vi "Main On Compile Action VI_Parse BC.vi"(7 "Autocreate Rx timestamp chans?":bool, 8 "error in":errorcluster, 10 "Channel Ref":u64, 11 "Device Item Ref in":T2 format="%.0x") -> (0 "error out":errorcluster, 2 "Channel Ref":u64, 3 "BC":T1 {"Acyclic Frames Trigger Channels Refs" format="%.0x"; "Command Channels Refs" format="%.0x"; "messages"."Timestamp Channel Data Reference" format="%.0x"; "messages"."Status Channel Data Refs" format="%.0x"; "messages"."Words Item Refs" format="%.0x"; "messages"."Words Block Data Refs"."Data Reference" format="%.0x"})   [LabVIEW 2020, in "Ballard 1553 System Explorer.lvlib"]
uses:
  Ballard 1553 System Explorer.lvlib
  <vilib>/NI VeriStand/Custom Device API/Custom Device Item Ref.ctl
  Shared/Controls and Global/RT BC.ctl
  Shared/Controls and Global/RT Message.ctl
  Shared/Controls and Global/RT messageType.ctl
  Shared/Controls and Global/RT CWD1.ctl
  Shared/Controls and Global/RT CWD2.ctl
  <vilib>/NI VeriStand/Custom Device API/Data Reference.ctl
  <vilib>/NI VeriStand/Custom Device API/Block Data Reference.ctl
  Shared/EncodeDecode/_typedefs/parameter_config_type.ctl
  Shared/EncodeDecode/_typedefs/parameter_config_type_type.ctl
  Shared/EncodeDecode/_typedefs/parameter_config_encoding_type.ctl
  Parse XML Ballard/Ballard_messageType.ctl
  Parse XML Ballard/Ballard_CWD1.ctl
  Parse XML Ballard/Ballard_CWD2.ctl
  <vilib>/NI VeriStand/Custom Device API/Data Access Type.ctl
  Shared/Controls and Global/Global.vi
  <vilib>/NI VeriStand/Custom Device Tools/Custom Device Utility Library/NI VeriStand - Search for Item by GUID.vi
  <vilib>/NI VeriStand/Custom Device API/Get Item Property (I32).vi
  <vilib>/NI VeriStand/Custom Device API/Get Item Property (String).vi
  <vilib>/NI VeriStand/Custom Device Tools/Custom Device Utility Library/NI VeriStand - Search for Item by Name.vi
  <vilib>/NI VeriStand/Custom Device Tools/Custom Device Utility Library/NI VeriStand - Search for All Items by GUID.vi
  <vilib>/NI VeriStand/Custom Device API/Get Item Property (Variant).vi
  <vilib>/NI VeriStand/Custom Device API/Get Item Property (U16).vi
  Shared/Ballard 1553 Shared.lvlib
  <vilib>/NI VeriStand/Custom Device Tools/Custom Device Utility Library/Custom Device Utility Library.lvlib
  <vilib>/NI VeriStand/Custom Device API/Custom Device API.lvlib
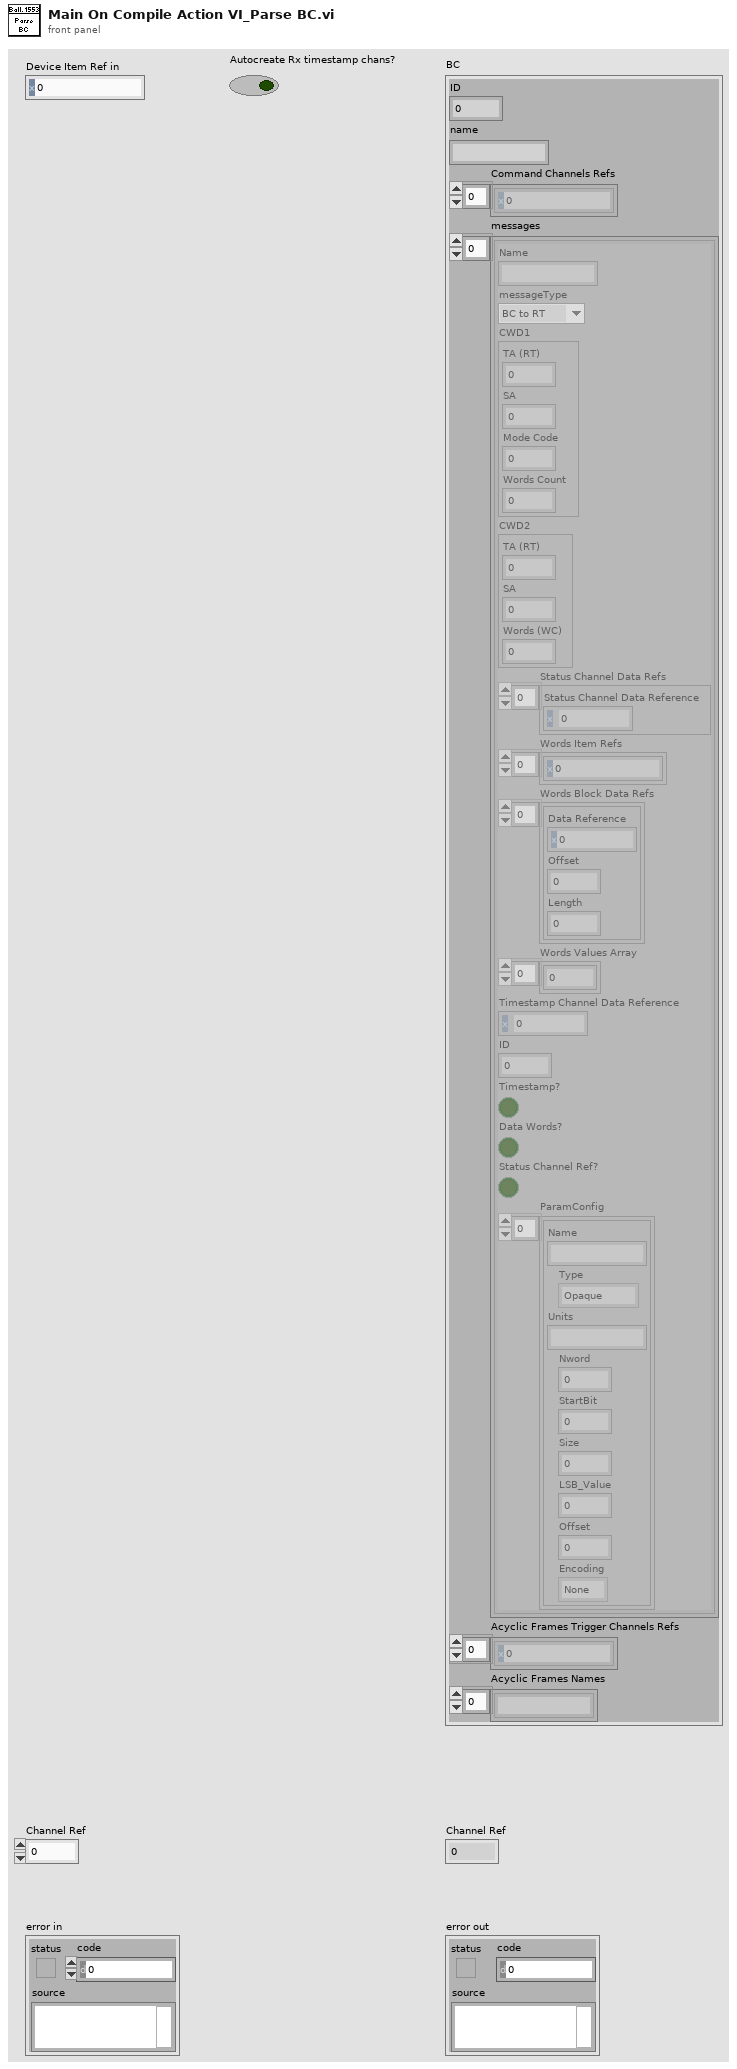
[diagram p1: front panel]
types:
  T1 = typedef "Ballard 1553 Shared.lvlib/RT BC.ctl" = cluster{"ID":i32, "name":string, "Command Channels Refs":T2[], "messages":T3[], "Acyclic Frames Trigger Channels Refs":T2[], "Acyclic Frames Names":string[]}
  T2 = typedef "Custom Device API.lvlib/Custom Device Item Ref.ctl" = u64
  T3 = typedef "Ballard 1553 Shared.lvlib/RT Message.ctl" = cluster{"Name":string, "messageType":T4, "CWD1":T5, "CWD2":T6, "Status Channel Data Refs":T7[], "Words Item Refs":T2[], "Words Block Data Refs":T8[], "Words Values Array":u16[], "Timestamp Channel Data Reference":T7, "ID":i32, "Timestamp?":bool, "Data Words?":bool, "Status Channel Ref?":bool, "ParamConfig":T9[]}
  T4 = typedef "Ballard 1553 Shared.lvlib/RT messageType.ctl" = enum16{"BC to RT", "RT to BC", "RT to RT", "MC (Rx)", "MC (Tx)"}
  T5 = typedef "Ballard 1553 Shared.lvlib/RT CWD1.ctl" = cluster{"TA (RT)":i8, "SA":i8, "Mode Code":i8, "Words Count":i8}
  T6 = typedef "Ballard 1553 Shared.lvlib/RT CWD2.ctl" = cluster{"TA (RT)":i8, "SA":i8, "Words (WC)":i8}
  T7 = typedef "Custom Device API.lvlib/Data Reference.ctl" = i32
  T8 = typedef "Custom Device API.lvlib/Block Data Reference.ctl" = cluster{"Data Reference":T7, "Offset":u64, "Length":u64}
  T9 = typedef "parameter_config_type.ctl" = cluster{"Name":string, "Type":T10, "Units":string, "Nword":i32, "StartBit":i32, "Size":i32, "LSB_Value":i32, "Offset":i32, "Encoding":T11}
  T10 = typedef "parameter_config_type_type.ctl" = enum16{"Opaque", "Enum", "Float", "Integer", "Bcd", "Bool"}
  T11 = typedef "parameter_config_encoding_type.ctl" = enum16{"None", "2-complement", "Unsigned"}
  T12 = typedef "Ballard 1553 System Explorer.lvlib/Ballard_CWD2.ctl" = cluster{"TA (RT)":i8, "SA":i8, "Words (WC)":i8}
  T13 = typedef "Ballard 1553 System Explorer.lvlib/Ballard_CWD1.ctl" = cluster{"TA (RT)":i8, "SA":i8, "Mode Code":i8, "Words Count":i8}
  T14 = typedef "Ballard 1553 System Explorer.lvlib/Ballard_messageType.ctl" = enum16{"BC to RT", "RT to BC", "RT to RT", "MC (Rx)", "MC (Tx)"}
  T15 = typedef "Custom Device API.lvlib/Data Access Type.ctl" = enum16{"Read", "Write"}
  T16 = typedef "Custom Device API.lvlib/Custom Device Item Info.ctl" = cluster{"Name":string, "Is Channel":bool, "GUID":string, "Is Waveform":bool}
  T17 = typedef "Custom Device API.lvlib/Custom Device Channel.ctl" = cluster{"Type":T18, "Units":string, "Default Value":dbl, "Faultable":bool, "Scalable":bool}
  T18 = typedef "Custom Device API.lvlib/Custom Device Channel Type.ctl" = enum16{"Input", "Output"}
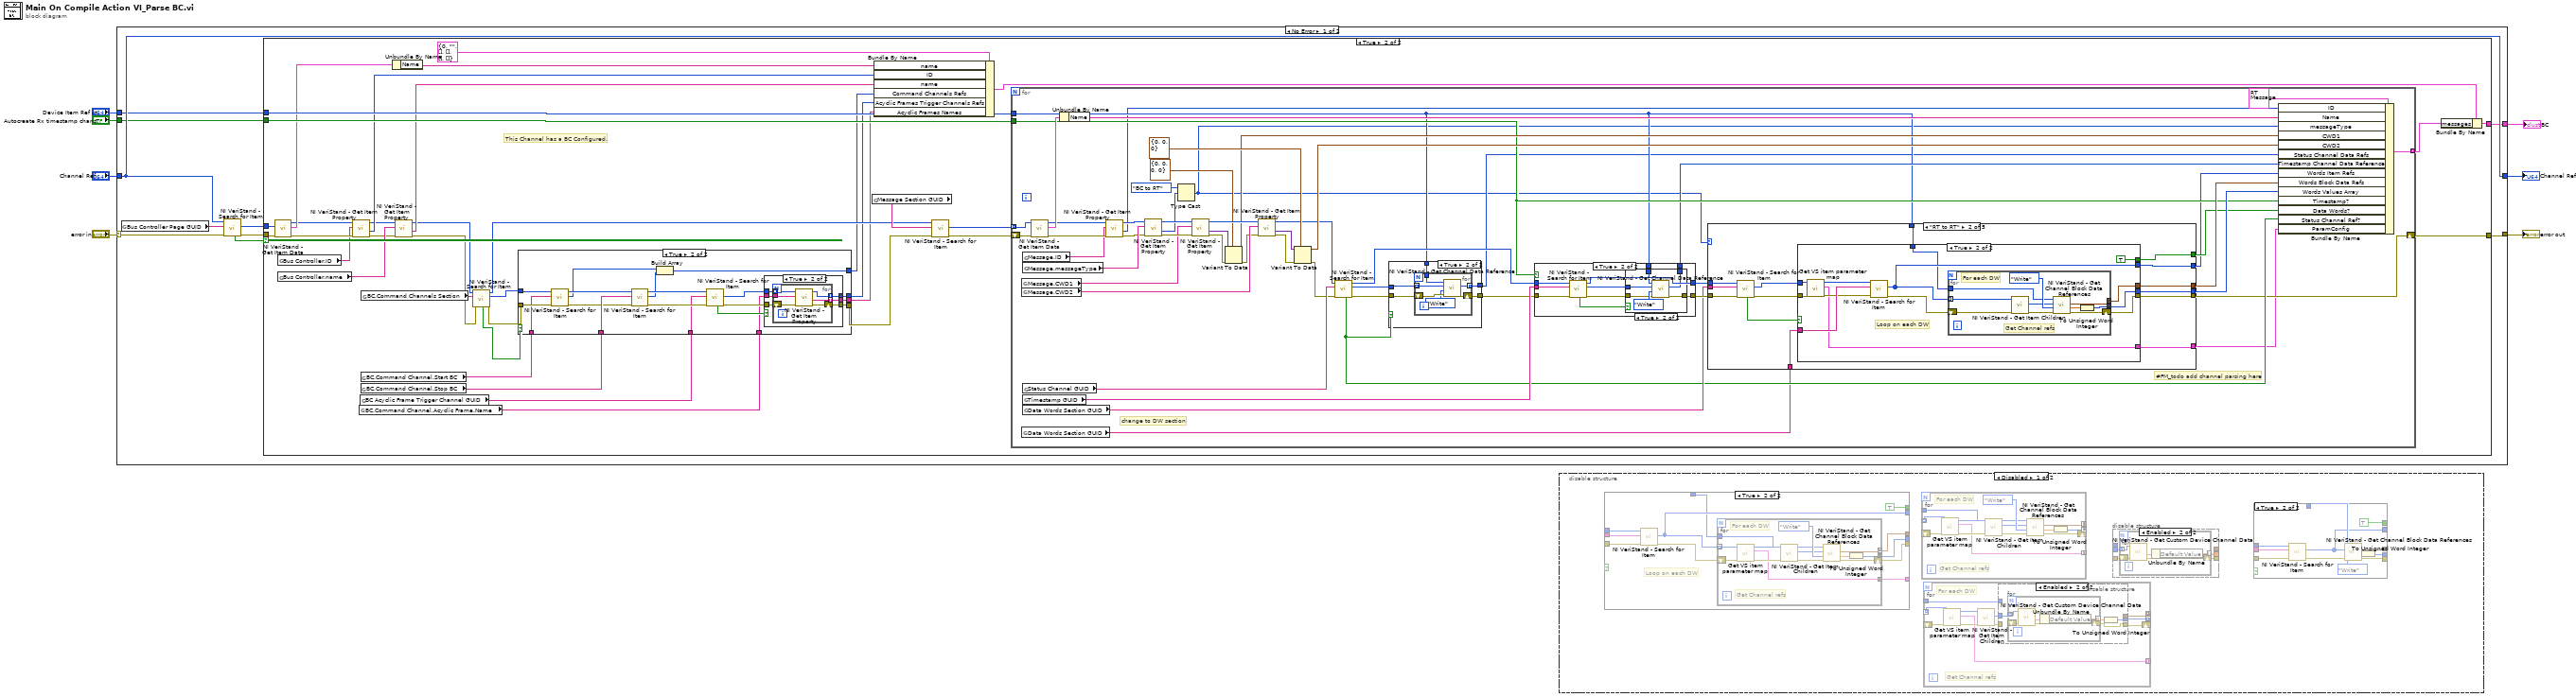
[diagram p0: block diagram]
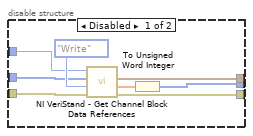
[diagram p2: hidden frame]
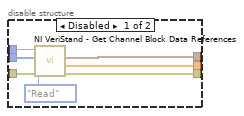
[diagram p3: hidden frame]
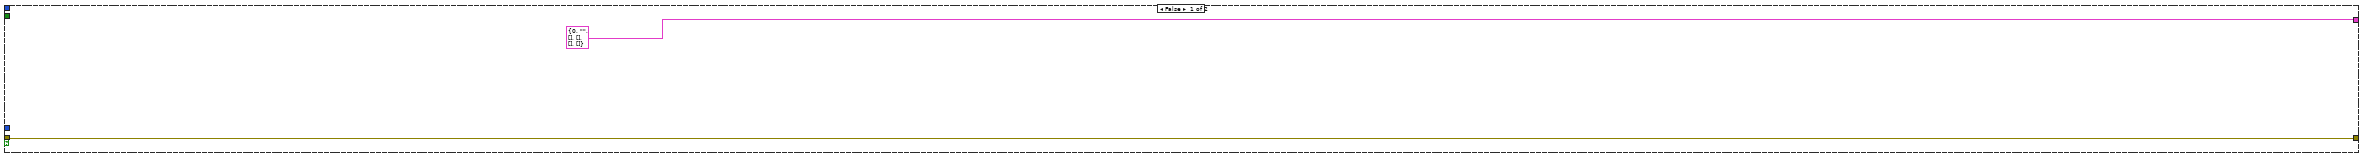
[diagram p7: hidden frame]
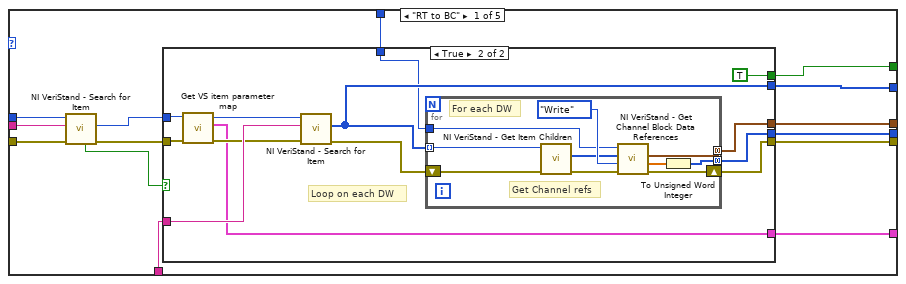
[diagram p11: hidden frame]
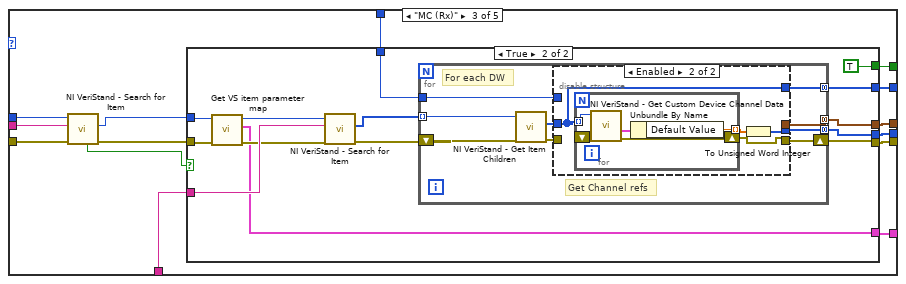
[diagram p14: hidden frame]
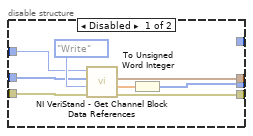
[diagram p16: hidden frame]
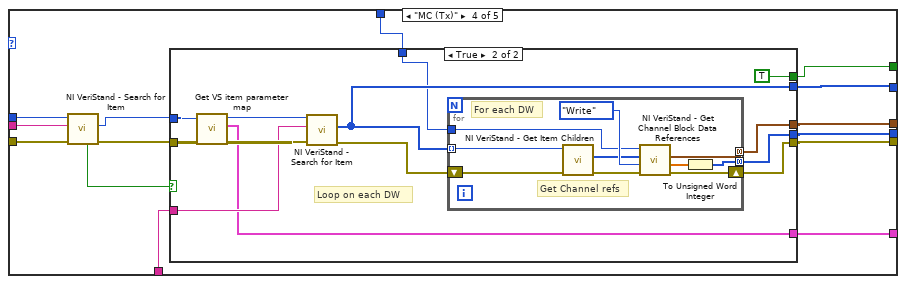
[diagram p17: hidden frame]
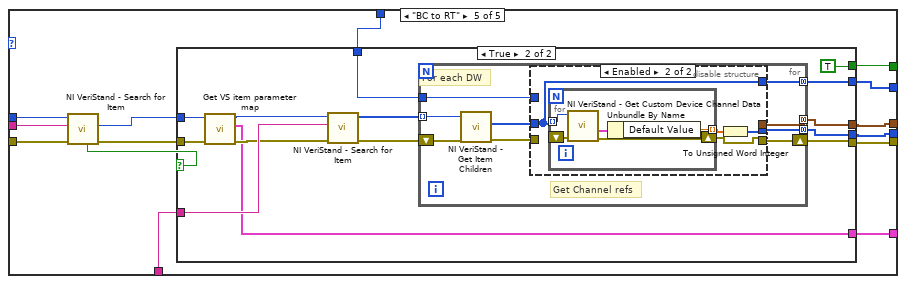
[diagram p19: hidden frame]
diagram:
  n1 = case shown="No Error" "error in" {
    selector: "error in" -> [w16 w401]
    tunnel: [w17 w401] -> w6
    tunnel: "Channel Ref" -> [w14 w400]
    tunnel: [w14 w400] -> w4
    tunnel: "Autocreate Rx timestamp chans?" -> [w10 _]
    tunnel: "Device Item Ref in" -> [w9 _]
    tunnel: [w8 T1 {"ID"=0, "name"="", "Command Channels Refs"=[], "messages"=[], "Acyclic Frames Trigger Channels Refs"=[], "Acyclic Frames Names"=[]} ("BC")] -> w1
    frame No Error {
      n2 = global read "Global.vi" "Bus Controller Page GUID"() -> (w15:string)
      n3 = call-poly <vilib>:"NI VeriStand - Search for Item.vi"("error in"=w16, "Item GUID"=w15, "Section Ref in"=w14) -> ("error out"=w13:errorcluster, "Item Ref"=w11:T2, "Found"=w12:bool)  [unwired: 5 in, 1 out]
      n4 = case shown="True" w12 {
        tunnel: w13 -> [w19 w39]
        tunnel: w11 -> [_ w40]
        tunnel: w10 -> [_ w53]
        tunnel: [w19 w52] -> w17
        tunnel: w9 -> [_ w51]
        tunnel: [T1 {"ID"=0, "name"="", "Command Channels Refs"=[], "messages"=[], "Acyclic Frames Trigger Channels Refs"=[], "Acyclic Frames Names"=[]} ("BC") w49] -> w8
        frame False {
        }
        frame True {
          # "This Channel has a BC Configured."
          n5 = call <vilib>:"NI VeriStand - Get Item Data.vi"("error in (no error)"=w39, "Item Ref in"=w40) -> ("error out"=w33:errorcluster, "Item Info"=w38:T16, "Item Ref out"=w34:T2)  [unwired: 6 in, 1 out]
          n6 = global read "Global.vi" "Bus Controller.ID"() -> (w32:string)
          n7 = global read "Global.vi" "Bus Controller.name"() -> (w29:string)
          n8 = call-poly <vilib>:"NI VeriStand - Get Item Property.vi"("error in (no error)"=w33, "Property Name"=w32, "Item Ref in"=w34) -> ("error out"=w28:errorcluster, "Value"=w31:i32, "Item Ref out"=w30:T2)  [unwired: 5 in, 1 out]
          n9 = global read "Global.vi" "BC.Command Channel.Acyclic Frame.Name"() -> (w22:string)
          n10 = global read "Global.vi" "BC Acyclic Frame Trigger Channel GUID"() -> (w23:string)
          n11 = global read "Global.vi" "BC.Command Channel.Start BC"() -> (w43:string)
          n12 = global read "Global.vi" "BC.Command Channel.Stop BC"() -> (w42:string)
          n13 = global read "Global.vi" "BC.Command Channels Section"() -> (w45:string)
          n14 = Unbundle By Name(w38) -> ("Name"=w36:string)
          n15 = call-poly <vilib>:"NI VeriStand - Get Item Property.vi"("error in (no error)"=w28, "Property Name"=w29, "Item Ref in"=w30) -> ("error out"=w27:errorcluster, "Value"=w26:string, "Item Ref out"=w24:T2)  [unwired: 5 in, 1 out]
          n16 = call-poly <vilib>:"NI VeriStand - Search for Item.vi"("error in"=w27, "Item Name"=w45, "Section Ref in"=w24) -> ("error out"=w46:errorcluster, "Item Ref"=w48:T2, "Section Ref out"=w41:T2, "Found"=w47:bool)  [unwired: 5 in]
          n17 = case shown="True" w47 {
            tunnel: w46 -> [w57 w76]
            tunnel: w48 -> [_ w75]
            tunnel: w43 -> [_ w74]
            tunnel: w42 -> [_ w73]
            tunnel: [w57 w61] -> w44
            tunnel: [_ w70] -> w25
            tunnel: [_ w60] -> w21
            tunnel: w23 -> [_ w68]
            tunnel: [_ w59] -> w20
            tunnel: w22 -> [_ w58]
            frame False {
            }
            frame True {
              n18 = call-poly <vilib>:"NI VeriStand - Search for Item.vi"("error in"=w76, "Item Name"=w74, "Section Ref in"=w75) -> ("error out"=w71:errorcluster, "Item Ref"=w66:T2, "Section Ref out"=w72:T2)  [unwired: 5 in, 1 out]
              n19 = call-poly <vilib>:"NI VeriStand - Search for Item.vi"("error in"=w71, "Item Name"=w73, "Section Ref in"=w72) -> ("error out"=w69:errorcluster, "Item Ref"=w65:T2, "Section Ref out"=w67:T2)  [unwired: 5 in, 1 out]
              n20 = Build Array(w66, w65) -> (w70:T2[])
              n21 = call-poly <vilib>:"NI VeriStand - Search for Item.vi"("error in"=w69, "Item GUID"=w68, "Section Ref in"=w67) -> ("error out"=w63:errorcluster, "Item Refs"=w62:T2[], "Found"=w64:bool)  [unwired: 5 in, 1 out]
              n22 = case shown="True" w64 {
                tunnel: w63 -> [w78 w83]
                tunnel: w62 -> [w77 w84]
                tunnel: [w78 w82] -> w61
                tunnel: [w77 w81] -> w60
                tunnel: [_ w80] -> w59
                tunnel: w58 -> [_ w79]
                frame False {
                }
                frame True {
                  n23 = for {
                    tunnel: w84 -> [w90] mode=indexing
                    shift-right: [w88] -> w82
                    shift-left: w83 -> [w89]
                    tunnel: [w87] -> w81 mode=indexing
                    tunnel: [w86] -> w80 mode=indexing
                    tunnel: w79 -> [w85]
                    n24 = call-poly <vilib>:"NI VeriStand - Get Item Property.vi"("error in (no error)"=w89, "Property Name"=w85, "Item Ref in"=w90) -> ("error out"=w88:errorcluster, "Value"=w86:string, "Item Ref out"=w87:T2)  [unwired: 5 in, 1 out]
                  }
                }
              }
            }
          }
          n25 = global read "Global.vi" "Message Section GUID"() -> (w56:string)
          n26 = Bundle By Name(cluster=T1 {"ID"=0, "name"="", "Command Channels Refs"=[], "messages"=[], "Acyclic Frames Trigger Channels Refs"=[], "Acyclic Frames Names"=[]} ("BC"), "name"=w36, "ID"=w31, "name"=w26, "Command Channels Refs"=w25, "Acyclic Frames Trigger Channels Refs"=w21, "Acyclic Frames Names"=w20) -> (w35:T1)
          n27 = call-poly <vilib>:"NI VeriStand - Search for Item.vi"("error in"=w44, "Item GUID"=w56, "Section Ref in"=w41) -> ("error out"=w55:errorcluster, "Item Refs"=w54:T2[])  [unwired: 5 in, 2 out]
          n28 = for {
            tunnel: w54 -> [w122] mode=indexing
            shift-right: [w94] -> w52
            shift-left: w55 -> [w123]
            tunnel: w53 -> [w106]
            tunnel: w51 -> [w98]
            tunnel: [w115] -> w50 mode=indexing
            # "change to DW section"
            # "#FM_todo add channel parsing here"
            n29 = global read "Global.vi" "Message.CWD1"() -> (w139:string)
            n30 = global read "Global.vi" "Message.CWD2"() -> (w138:string)
            n31 = global read "Global.vi" "Data Words Section GUID"() -> (w93:string)
            n32 = global read "Global.vi" "Message.ID"() -> (w109:string)
            n33 = global read "Global.vi" "Message.messageType"() -> (w140:string)
            n34 = global read "Global.vi" "Status Channel GUID"() -> (w128:string)
            n35 = global read "Global.vi" "Timestamp GUID"() -> (w127:string)
            n36 = global read "Global.vi" "Data Words Section GUID"() -> (w124:string)
            n37 = call <vilib>:"NI VeriStand - Get Item Data.vi"("error in (no error)"=w123, "Item Ref in"=w122) -> ("error out"=w110:errorcluster, "Item Info"=w121:T16, "Item Ref out"=w111:T2)  [unwired: 6 in, 1 out]
            n38 = Unbundle By Name(w121) -> ("Name"=w120:string)
            n39 = call-poly <vilib>:"NI VeriStand - Get Item Property.vi"("error in (no error)"=w110, "Property Name"=w109, "Item Ref in"=w111) -> ("error out"=w108:errorcluster, "Value"=w95:i32, "Item Ref out"=w107:T2)  [unwired: 5 in, 1 out]
            n40 = call-poly <vilib>:"NI VeriStand - Get Item Property.vi"("error in (no error)"=w108, "Property Name"=w140, "Item Ref in"=w107) -> ("error out"=w143:errorcluster, "Value"=w132:u16, "Item Ref out"=w141:T2)  [unwired: 5 in, 1 out]
            n41 = Type Cast(type=Ballard_messageType."BC to RT" ("messageType"), x=w132) -> (*(type *) &x=w96:T14)
            n42 = call-poly <vilib>:"NI VeriStand - Get Item Property.vi"("error in (no error)"=w143, "Property Name"=w139, "Item Ref in"=w141) -> ("error out"=w137:errorcluster, "Value"=w134:variant, "Item Ref out"=w142:T2)  [unwired: 5 in, 1 out]
            n43 = Variant To Data(error in=w137, type=T13 {"TA (RT)"=0, "SA"=0, "Mode Code"=0, "Words Count"=0} ("CWD1"), Variant=w134) -> (data=w119:T13, error out=w135:errorcluster)
            n44 = call-poly <vilib>:"NI VeriStand - Get Item Property.vi"("error in (no error)"=w135, "Property Name"=w138, "Item Ref in"=w142) -> ("error out"=w136:errorcluster, "Value"=w133:variant, "Item Ref out"=w114:T2)  [unwired: 5 in, 1 out]
            n45 = Variant To Data(error in=w136, type=T12 {"TA (RT)"=0, "SA"=0, "Words (WC)"=0} ("CWD1"), Variant=w133) -> (data=w118:T12, error out=w113:errorcluster)
            n46 = call-poly <vilib>:"NI VeriStand - Search for Item.vi"("error in"=w113, "Item GUID"=w128, "Section Ref in"=w114) -> ("error out"=w102:errorcluster, "Item Refs"=w100:T2[], "Section Ref out"=w99:T2, "Found"=w103:bool)  [unwired: 5 in]
            n47 = case shown="True" w103 {
              tunnel: w102 -> [w144 w149]
              tunnel: [w144 w148] -> w101
              tunnel: w100 -> [_ w146]
              tunnel: w98 -> [_ w147]
              tunnel: [_ w145] -> w97
              frame False {
              }
              frame True {
                n48 = for {
                  tunnel: w147 -> [w153]
                  shift-right: [w154] -> w148
                  shift-left: w149 -> [w155]
                  tunnel: w146 -> [w151] mode=indexing
                  tunnel: [w150] -> w145 mode=indexing
                  n49 = call <vilib>:"NI VeriStand - Get Channel Data Reference.vi"("error in (no error)"=w155, "Access"=Data_Access_Type."Write", "Channel Ref in"=w151, "Device Ref in"=w153) -> ("error out"=w154:errorcluster, "Channel Data Reference"=w150:T7)  [unwired: 5 in, 1 out]
                }
              }
            }
            n50 = case shown="True" w106 {
              tunnel: w99 -> [w380 w391]
              tunnel: w101 -> [w381 w390]
              tunnel: [w381 w388] -> w126
              tunnel: w127 -> [_ w389]
              tunnel: [w380 w386] -> w125
              tunnel: w98 -> [_ w385]
              tunnel: [_ w383] -> w104
              frame False {
              }
              frame True {
                n51 = call-poly <vilib>:"NI VeriStand - Search for Item.vi"("error in"=w390, "Item GUID"=w389, "Section Ref in"=w391) -> ("error out"=w387:errorcluster, "Item Ref"=w384:T2, "Section Ref out"=w386:T2, "Found"=w382:bool)  [unwired: 5 in]
                n52 = case shown="True" w382 {
                  tunnel: [w392 w397] -> w388
                  tunnel: w387 -> [w392 w396]
                  tunnel: w385 -> [_ w395]
                  tunnel: w384 -> [_ w394]
                  tunnel: [_ w393] -> w383
                  frame False {
                  }
                  frame True {
                    n53 = call <vilib>:"NI VeriStand - Get Channel Data Reference.vi"("error in (no error)"=w396, "Access"=Data_Access_Type."Write", "Channel Ref in"=w394, "Device Ref in"=w395) -> ("error out"=w397:errorcluster, "Channel Data Reference"=w393:T7)  [unwired: 5 in, 1 out]
                  }
                }
              }
            }
            n54 = case shown="\"RT to RT\"" w96 {
              tunnel: w126 -> [w169 w207 w245 w300 w338]
              tunnel: w125 -> [w168 w206 w244 w299 w337]
              tunnel: w124 -> [w167 w205 w243 w298 w336]
              tunnel: w93 -> [w164 w203 w239 w295 w333]
              tunnel: [w163 w197 w238 w290 w328] -> w94
              tunnel: w98 -> [w162 w200 w237 w293 w331]
              tunnel: [w161 w198 w236 w292 w329] -> w117
              tunnel: [w160 w199 w235 w291 w330] -> w116
              tunnel: [w159 w196 w233 w288 w326] -> w92
              tunnel: [w158 w195 w234 w289 w327] -> w105
              tunnel: [w156 w194 w232 w287 w335] -> w91
              frame "RT to BC" {
                n55 = call-poly <vilib>:"NI VeriStand - Search for Item.vi"("error in"=w169, "Item GUID"=w167, "Section Ref in"=w168) -> ("error out"=w166:errorcluster, "Item Ref"=w165:T2, "Found"=w157:bool)  [unwired: 5 in, 1 out]
                n56 = case shown="True" w157 {
                  tunnel: w166 -> [w170 w174]
                  tunnel: w165 -> [_ w175]
                  tunnel: w164 -> [_ w183]
                  tunnel: [w170 w176] -> w163
                  tunnel: w162 -> [_ w179]
                  tunnel: [_ w180] -> w159
                  tunnel: [_ w177] -> w161
                  tunnel: [_ w178] -> w160
                  tunnel: [_ TRUE] -> w158
                  tunnel: [_ w171] -> w156
                  frame False {
                  }
                  frame True {
                    # "Loop on each DW"
                    n57 = call "Get VS item parameter map.vi"("error in (no error)"=w174, "Iten refs in"=w175) -> ("error out"=w173:errorcluster, "param config out"=w171:T9[], "Iten refs out"=w172:T2)  [unwired: 6 in, 1 out]
                    n58 = call-poly <vilib>:"NI VeriStand - Search for Item.vi"("error in"=w173, "Item GUID"=w183, "Section Ref in"=w172) -> ("error out"=w181:errorcluster, "Item Refs"=w180:T2[])  [unwired: 5 in, 2 out]
                    n59 = for {
                      shift-right: [w188] -> w176
                      shift-left: w181 -> [w186]
                      tunnel: w180 -> [w187] mode=indexing
                      tunnel: w179 -> [w191]
                      tunnel: [w190] -> w178 mode=concatenating
                      tunnel: [w189] -> w177 mode=concatenating
                      # "Get Channel refs"
                      # "For each DW"
                      n60 = call <vilib>:"NI VeriStand - Get Item Children.vi"("error in (no error)"=w186, "Item Ref in"=w187) -> ("error out"=w184:errorcluster, "Child Refs"=w185:T2[])  [unwired: 6 in, 2 out]
                      n61 = call <vilib>:"NI VeriStand - Get Channel Block Data References.vi"("error in (no error)"=w184, "Access"=Data_Access_Type."Write", "Channel Refs"=w185, "Device Ref in"=w191) -> ("error out"=w188:errorcluster, "Values Array"=w193:dbl[], "Block Data Refs"=w189:T8[])  [unwired: 4 in, 1 out]
                      n62 = To Unsigned Word Integer(number=w193) -> (unsigned 16bit integer=w190:u16[])
                    }
                  }
                }
              }
              frame "RT to RT" {
                n63 = call-poly <vilib>:"NI VeriStand - Search for Item.vi"("error in"=w207, "Item GUID"=w205, "Section Ref in"=w206) -> ("error out"=w202:errorcluster, "Item Ref"=w204:T2, "Found"=w201:bool)  [unwired: 5 in, 1 out]
                n64 = case shown="True" w201 {
                  tunnel: w202 -> [w208 w212]
                  tunnel: w204 -> [_ w213]
                  tunnel: w203 -> [_ w221]
                  tunnel: [w208 w214] -> w197
                  tunnel: w200 -> [_ w217]
                  tunnel: [_ w218] -> w196
                  tunnel: [_ w215] -> w198
                  tunnel: [_ w216] -> w199
                  tunnel: [_ TRUE] -> w195
                  tunnel: [_ w209] -> w194
                  frame False {
                  }
                  frame True {
                    # "Loop on each DW"
                    n65 = call "Get VS item parameter map.vi"("error in (no error)"=w212, "Iten refs in"=w213) -> ("error out"=w211:errorcluster, "param config out"=w209:T9[], "Iten refs out"=w210:T2)  [unwired: 6 in, 1 out]
                    n66 = call-poly <vilib>:"NI VeriStand - Search for Item.vi"("error in"=w211, "Item GUID"=w221, "Section Ref in"=w210) -> ("error out"=w219:errorcluster, "Item Refs"=w218:T2[])  [unwired: 5 in, 2 out]
                    n67 = for {
                      shift-right: [w226] -> w214
                      shift-left: w219 -> [w224]
                      tunnel: w218 -> [w225] mode=indexing
                      tunnel: w217 -> [w229]
                      tunnel: [w228] -> w216 mode=concatenating
                      tunnel: [w227] -> w215 mode=concatenating
                      # "Get Channel refs"
                      # "For each DW"
                      n68 = call <vilib>:"NI VeriStand - Get Item Children.vi"("error in (no error)"=w224, "Item Ref in"=w225) -> ("error out"=w222:errorcluster, "Child Refs"=w223:T2[])  [unwired: 6 in, 2 out]
                      n69 = call <vilib>:"NI VeriStand - Get Channel Block Data References.vi"("error in (no error)"=w222, "Access"=Data_Access_Type."Write", "Channel Refs"=w223, "Device Ref in"=w229) -> ("error out"=w226:errorcluster, "Values Array"=w231:dbl[], "Block Data Refs"=w227:T8[])  [unwired: 4 in, 1 out]
                      n70 = To Unsigned Word Integer(number=w231) -> (unsigned 16bit integer=w228:u16[])
                    }
                  }
                }
              }
              frame "MC (Rx)" {
                n71 = call-poly <vilib>:"NI VeriStand - Search for Item.vi"("error in"=w245, "Item GUID"=w243, "Section Ref in"=w244) -> ("error out"=w242:errorcluster, "Item Ref"=w240:T2, "Found"=w241:bool)  [unwired: 5 in, 1 out]
                n72 = case shown="True" w241 {
                  tunnel: w242 -> [w246 w251]
                  tunnel: w240 -> [_ w250]
                  tunnel: w239 -> [_ w260]
                  tunnel: [w246 w256] -> w238
                  tunnel: w237 -> [_ w253]
                  tunnel: [_ w255] -> w236
                  tunnel: [_ w254] -> w235
                  tunnel: [_ TRUE] -> w234
                  tunnel: [_ w252] -> w233
                  tunnel: [_ w247] -> w232
                  frame False {
                  }
                  frame True {
                    n73 = call "Get VS item parameter map.vi"("error in (no error)"=w251, "Iten refs in"=w250) -> ("error out"=w248:errorcluster, "param config out"=w247:T9[], "Iten refs out"=w249:T2)  [unwired: 6 in, 1 out]
                    n74 = call-poly <vilib>:"NI VeriStand - Search for Item.vi"("error in"=w248, "Item GUID"=w260, "Section Ref in"=w249) -> ("error out"=w257:errorcluster, "Item Refs"=w258:T2[])  [unwired: 5 in, 2 out]
                    n75 = for {
                      shift-right: [w266] -> w256
                      shift-left: w257 -> [w264]
                      tunnel: w258 -> [w265] mode=indexing
                      tunnel: w253 -> [w269]
                      tunnel: [w268] -> w254 mode=concatenating
                      tunnel: [w267] -> w255 mode=concatenating
                      tunnel: [w261] -> w252 mode=concatenating
                      # "Get Channel refs"
                      # "For each DW"
                      n76 = call <vilib>:"NI VeriStand - Get Item Children.vi"("error in (no error)"=w264, "Item Ref in"=w265) -> ("error out"=w262:errorcluster, "Child Refs"=w263:T2[])  [unwired: 6 in, 2 out]
                      n77 = disable-structure shown="Enabled" {
                        disable-tunnel: w269 -> [w275 _]
                        disable-tunnel: [w274 w280] -> w268
                        disable-tunnel: [w273 _] -> w267
                        disable-tunnel: [w272 w279] -> w266
                        disable-tunnel: w263 -> [w271 w278]
                        disable-tunnel: w262 -> [w270 _]
                        disable-tunnel: [_ w278] -> w261
                        frame Disabled {
                          n78 = call <vilib>:"NI VeriStand - Get Channel Block Data References.vi"("error in (no error)"=w270, "Access"=Data_Access_Type."Write", "Channel Refs"=w271, "Device Ref in"=w275) -> ("error out"=w272:errorcluster, "Values Array"=w277:dbl[], "Block Data Refs"=w273:T8[])  [unwired: 4 in, 1 out]
                          n79 = To Unsigned Word Integer(number=w277) -> (unsigned 16bit integer=w274:u16[])
                        }
                        frame Enabled {
                          n80 = for {
                            tunnel: [w282] -> w281 mode=indexing
                            shift-right: [w283] -> w279
                            shift-left: _ -> [w286]
                            tunnel: w278 -> [w284] mode=indexing
                            n81 = call <vilib>:"NI VeriStand - Get Custom Device Channel Data.vi"("error in (no error)"=w286, "Channel Ref in"=w284) -> ("error out"=w283:errorcluster, "Channel"=w285:T17)  [unwired: 4 in, 4 out]
                            n82 = Unbundle By Name(w285) -> ("Default Value"=w282:dbl)
                          }
                          n83 = To Unsigned Word Integer(number=w281) -> (unsigned 16bit integer=w280:u16[])
                        }
                      }
                    }
                  }
                }
              }
              frame "MC (Tx)" {
                n84 = call-poly <vilib>:"NI VeriStand - Search for Item.vi"("error in"=w300, "Item GUID"=w298, "Section Ref in"=w299) -> ("error out"=w297:errorcluster, "Item Ref"=w294:T2, "Found"=w296:bool)  [unwired: 5 in, 1 out]
                n85 = case shown="True" w296 {
                  tunnel: w297 -> [w301 w305]
                  tunnel: w294 -> [_ w306]
                  tunnel: w295 -> [_ w314]
                  tunnel: [w301 w307] -> w290
                  tunnel: w293 -> [_ w310]
                  tunnel: [_ w311] -> w288
                  tunnel: [_ w308] -> w292
                  tunnel: [_ w309] -> w291
                  tunnel: [_ TRUE] -> w289
                  tunnel: [_ w302] -> w287
                  frame False {
                  }
                  frame True {
                    # "Loop on each DW"
                    n86 = call "Get VS item parameter map.vi"("error in (no error)"=w305, "Iten refs in"=w306) -> ("error out"=w303:errorcluster, "param config out"=w302:T9[], "Iten refs out"=w304:T2)  [unwired: 6 in, 1 out]
                    n87 = call-poly <vilib>:"NI VeriStand - Search for Item.vi"("error in"=w303, "Item GUID"=w314, "Section Ref in"=w304) -> ("error out"=w312:errorcluster, "Item Refs"=w311:T2[])  [unwired: 5 in, 2 out]
                    n88 = for {
                      shift-right: [w319] -> w307
                      shift-left: w312 -> [w317]
                      tunnel: w311 -> [w318] mode=indexing
                      tunnel: w310 -> [w322]
                      tunnel: [w321] -> w309 mode=concatenating
                      tunnel: [w320] -> w308 mode=concatenating
                      # "Get Channel refs"
                      # "For each DW"
                      n89 = call <vilib>:"NI VeriStand - Get Item Children.vi"("error in (no error)"=w317, "Item Ref in"=w318) -> ("error out"=w315:errorcluster, "Child Refs"=w316:T2[])  [unwired: 6 in, 2 out]
                      n90 = call <vilib>:"NI VeriStand - Get Channel Block Data References.vi"("error in (no error)"=w315, "Access"=Data_Access_Type."Write", "Channel Refs"=w316, "Device Ref in"=w322) -> ("error out"=w319:errorcluster, "Values Array"=w324:dbl[], "Block Data Refs"=w320:T8[])  [unwired: 4 in, 1 out]
                      n91 = To Unsigned Word Integer(number=w324) -> (unsigned 16bit integer=w321:u16[])
                    }
                  }
                }
              }
              frame "BC to RT" {
                n92 = call-poly <vilib>:"NI VeriStand - Search for Item.vi"("error in"=w338, "Item GUID"=w336, "Section Ref in"=w337) -> ("error out"=w334:errorcluster, "Item Ref"=w332:T2, "Found"=w325:bool)  [unwired: 5 in, 1 out]
                n93 = case shown="True" w325 {
                  tunnel: w334 -> [w339 w343]
                  tunnel: w332 -> [_ w344]
                  tunnel: w333 -> [_ w353]
                  tunnel: [w339 w349] -> w328
                  tunnel: w331 -> [_ w346]
                  tunnel: [_ w348] -> w329
                  tunnel: [_ w347] -> w330
                  tunnel: [_ TRUE] -> w327
                  tunnel: [_ w340] -> w335
                  tunnel: [_ w345] -> w326
                  frame False {
                  }
                  frame True {
                    n94 = call "Get VS item parameter map.vi"("error in (no error)"=w343, "Iten refs in"=w344) -> ("error out"=w342:errorcluster, "param config out"=w340:T9[], "Iten refs out"=w341:T2)  [unwired: 6 in, 1 out]
                    n95 = call-poly <vilib>:"NI VeriStand - Search for Item.vi"("error in"=w342, "Item GUID"=w353, "Section Ref in"=w341) -> ("error out"=w350:errorcluster, "Item Refs"=w351:T2[])  [unwired: 5 in, 2 out]
                    n96 = for {
                      shift-right: [w359] -> w349
                      shift-left: w350 -> [w357]
                      tunnel: w351 -> [w358] mode=indexing
                      tunnel: w346 -> [w362]
                      tunnel: [w361] -> w347 mode=concatenating
                      tunnel: [w360] -> w348 mode=concatenating
                      tunnel: [w354] -> w345 mode=concatenating
                      # "Get Channel refs"
                      # "For each DW"
                      n97 = call <vilib>:"NI VeriStand - Get Item Children.vi"("error in (no error)"=w357, "Item Ref in"=w358) -> ("error out"=w355:errorcluster, "Child Refs"=w356:T2[])  [unwired: 6 in, 2 out]
                      n98 = disable-structure shown="Enabled" {
                        disable-tunnel: w362 -> [w368 _]
                        disable-tunnel: [w367 w373] -> w361
                        disable-tunnel: [w366 _] -> w360
                        disable-tunnel: [w365 w372] -> w359
                        disable-tunnel: w356 -> [w364 w371]
                        disable-tunnel: w355 -> [w363 _]
                        disable-tunnel: [_ w371] -> w354
                        frame Disabled {
                          n99 = call <vilib>:"NI VeriStand - Get Channel Block Data References.vi"("error in (no error)"=w363, "Access"=Data_Access_Type."Write", "Channel Refs"=w364, "Device Ref in"=w368) -> ("error out"=w365:errorcluster, "Values Array"=w370:dbl[], "Block Data Refs"=w366:T8[])  [unwired: 4 in, 1 out]
                          n100 = To Unsigned Word Integer(number=w370) -> (unsigned 16bit integer=w367:u16[])
                        }
                        frame Enabled {
                          n101 = for {
                            tunnel: [w375] -> w374 mode=indexing
                            shift-right: [w376] -> w372
                            shift-left: _ -> [w379]
                            tunnel: w371 -> [w377] mode=indexing
                            n102 = call <vilib>:"NI VeriStand - Get Custom Device Channel Data.vi"("error in (no error)"=w379, "Channel Ref in"=w377) -> ("error out"=w376:errorcluster, "Channel"=w378:T17)  [unwired: 4 in, 4 out]
                            n103 = Unbundle By Name(w378) -> ("Default Value"=w375:dbl)
                          }
                          n104 = To Unsigned Word Integer(number=w374) -> (unsigned 16bit integer=w373:u16[])
                        }
                      }
                    }
                  }
                }
              }
            }
            n105 = Bundle By Name(cluster=T3 {"Name"="", "messageType"=enum."BC to RT", "CWD1"={"TA (RT)"=0, "SA"=0, "Mode Code"=0, "Words Count"=0}, "CWD2"={"TA (RT)"=0, "SA"=0, "Words (WC)"=0}, "Status Channel Data Refs"=[], "Words Item Refs"=[], "Words Block Data Refs"=[], "Words Values Array"=[], "Timestamp Channel Data Reference"=0, "ID"=0, "Timestamp?"=FALSE, "Data Words?"=FALSE, "Status Channel Ref?"=FALSE, "ParamConfig"=[]} ("output cluster"), "ID"=w95, "Name"=w120, "messageType"=w96, "CWD1"=w119, "CWD2"=w118, "Status Channel Data Refs"=w97, "Timestamp Channel Data Reference"=w104, "Words Item Refs"=w92, "Words Block Data Refs"=w117, "Words Values Array"=w116, "Timestamp?"=w106, "Data Words?"=w105, "Status Channel Ref?"=w103, "ParamConfig"=w91) -> (w115:T3)
          }
          n106 = Bundle By Name(cluster=w35, "messages"=w50) -> (w49:T1)
        }
      }
    }
    frame Error {
    }
  }
  "error out" <- w6
  "Channel Ref" <- w4
  "BC" <- w1
  n107 = disable-structure shown="Disabled" {
    frame Disabled {
      n108 = case shown="True" {
        selector: _ -> [_ _]
        tunnel: _ -> [w472 w481]
        tunnel: _ -> [_ w483]
        tunnel: _ -> [_ w482]
        tunnel: [w472 w474] -> _
        tunnel: _ -> [_ w477]
        tunnel: [_ w478] -> _
        tunnel: [_ w475] -> _
        tunnel: [_ w476] -> _
        tunnel: [_ TRUE] -> _
        tunnel: [_ w473] -> _
        frame False {
        }
        frame True {
          # "Loop on each DW"
          n109 = call-poly <vilib>:"NI VeriStand - Search for Item.vi"("error in"=w481, "Item GUID"=w482, "Section Ref in"=w483) -> ("error out"=w479:errorcluster, "Item Refs"=w478:T2[])  [unwired: 5 in, 2 out]
          n110 = for {
            shift-right: [w491] -> w474
            shift-left: w479 -> [w489]
            tunnel: w478 -> [w490] mode=indexing
            tunnel: w477 -> [w494]
            tunnel: [w493] -> w476 mode=concatenating
            tunnel: [w492] -> w475 mode=concatenating
            tunnel: [w484] -> w473 mode=concatenating
            # "Get Channel refs"
            # "For each DW"
            n111 = call "Get VS item parameter map.vi"("error in (no error)"=w489, "Iten refs in"=w490) -> ("error out"=w487:errorcluster, "param config out"=w484:T9[], "Iten refs out"=w488:T2)  [unwired: 6 in, 1 out]
            n112 = call <vilib>:"NI VeriStand - Get Item Children.vi"("error in (no error)"=w487, "Item Ref in"=w488) -> ("error out"=w485:errorcluster, "Child Refs"=w486:T2[])  [unwired: 6 in, 2 out]
            n113 = call <vilib>:"NI VeriStand - Get Channel Block Data References.vi"("error in (no error)"=w485, "Access"=Data_Access_Type."Write", "Channel Refs"=w486, "Device Ref in"=w494) -> ("error out"=w491:errorcluster, "Values Array"=w496:dbl[], "Block Data Refs"=w492:T8[])  [unwired: 4 in, 1 out]
            n114 = To Unsigned Word Integer(number=w496) -> (unsigned 16bit integer=w493:u16[])
          }
        }
      }
      n115 = for {
        shift-right: [w453] -> _
        shift-left: _ -> [w451]
        tunnel: _ -> [w452] mode=indexing
        tunnel: _ -> [w456]
        tunnel: [w455] -> _ mode=concatenating
        tunnel: [w454] -> _ mode=concatenating
        tunnel: [w446] -> _ mode=concatenating
        # "Get Channel refs"
        # "For each DW"
        n116 = call "Get VS item parameter map.vi"("error in (no error)"=w451, "Iten refs in"=w452) -> ("error out"=w449:errorcluster, "param config out"=w446:T9[], "Iten refs out"=w450:T2)  [unwired: 6 in, 1 out]
        n117 = call <vilib>:"NI VeriStand - Get Item Children.vi"("error in (no error)"=w449, "Item Ref in"=w450) -> ("error out"=w447:errorcluster, "Child Refs"=w448:T2[])  [unwired: 6 in, 2 out]
        n118 = call <vilib>:"NI VeriStand - Get Channel Block Data References.vi"("error in (no error)"=w447, "Access"=Data_Access_Type."Write", "Channel Refs"=w448, "Device Ref in"=w456) -> ("error out"=w453:errorcluster, "Values Array"=w458:dbl[], "Block Data Refs"=w454:T8[])  [unwired: 4 in, 1 out]
        n119 = To Unsigned Word Integer(number=w458) -> (unsigned 16bit integer=w455:u16[])
      }
      n120 = for {
        shift-right: [w409] -> _
        shift-left: _ -> [w407]
        tunnel: _ -> [w408] mode=indexing
        tunnel: _ -> [w412]
        tunnel: [w411] -> _ mode=concatenating
        tunnel: [w410] -> _ mode=concatenating
        tunnel: [w402] -> _ mode=concatenating
        # "Get Channel refs"
        # "For each DW"
        n121 = call "Get VS item parameter map.vi"("error in (no error)"=w407, "Iten refs in"=w408) -> ("error out"=w405:errorcluster, "param config out"=w402:T9[], "Iten refs out"=w406:T2)  [unwired: 6 in, 1 out]
        n122 = call <vilib>:"NI VeriStand - Get Item Children.vi"("error in (no error)"=w405, "Item Ref in"=w406) -> ("error out"=w403:errorcluster, "Child Refs"=w404:T2[])  [unwired: 6 in, 2 out]
        n123 = disable-structure shown="Enabled" {
          disable-tunnel: w412 -> [w418 _]
          disable-tunnel: [w417 w423] -> w411
          disable-tunnel: [w416 _] -> w410
          disable-tunnel: [w415 w422] -> w409
          disable-tunnel: w404 -> [w414 w421]
          disable-tunnel: w403 -> [w413 _]
          frame Disabled {
            n124 = call <vilib>:"NI VeriStand - Get Channel Block Data References.vi"("error in (no error)"=w413, "Access"=Data_Access_Type."Write", "Channel Refs"=w414, "Device Ref in"=w418) -> ("error out"=w415:errorcluster, "Values Array"=w420:dbl[], "Block Data Refs"=w416:T8[])  [unwired: 4 in, 1 out]
            n125 = To Unsigned Word Integer(number=w420) -> (unsigned 16bit integer=w417:u16[])
          }
          frame Enabled {
            n126 = for {
              tunnel: [w425] -> w424 mode=indexing
              shift-right: [w426] -> w422
              shift-left: _ -> [w429]
              tunnel: w421 -> [w427] mode=indexing
              n127 = call <vilib>:"NI VeriStand - Get Custom Device Channel Data.vi"("error in (no error)"=w429, "Channel Ref in"=w427) -> ("error out"=w426:errorcluster, "Channel"=w428:T17)  [unwired: 4 in, 4 out]
              n128 = Unbundle By Name(w428) -> ("Default Value"=w425:dbl)
            }
            n129 = To Unsigned Word Integer(number=w424) -> (unsigned 16bit integer=w423:u16[])
          }
        }
      }
      n130 = disable-structure shown="Enabled" {
        disable-tunnel: _ -> [w436 w439]
        disable-tunnel: [w435 w438] -> _
        disable-tunnel: _ -> [w434 _]
        disable-tunnel: _ -> [w432 w440]
        disable-tunnel: [w431 _] -> _
        disable-tunnel: [w430 w437] -> _
        frame Disabled {
          n131 = call <vilib>:"NI VeriStand - Get Channel Block Data References.vi"("error in (no error)"=w436, "Access"=Data_Access_Type."Read", "Channel Refs"=w432, "Device Ref in"=w434) -> ("error out"=w435:errorcluster, "Values Array"=w430:dbl[], "Block Data Refs"=w431:T8[])  [unwired: 4 in, 1 out]
        }
        frame Enabled {
          n132 = for {
            tunnel: [w441] -> w437 mode=indexing
            shift-right: [w442] -> w438
            shift-left: w439 -> [w445]
            tunnel: w440 -> [w443] mode=indexing
            n133 = call <vilib>:"NI VeriStand - Get Custom Device Channel Data.vi"("error in (no error)"=w445, "Channel Ref in"=w443) -> ("error out"=w442:errorcluster, "Channel"=w444:T17)  [unwired: 4 in, 4 out]
            n134 = Unbundle By Name(w444) -> ("Default Value"=w441:dbl)
          }
        }
      }
      n135 = case shown="True" {
        selector: _ -> [_ _]
        tunnel: _ -> [w459 w469]
        tunnel: _ -> [_ w471]
        tunnel: _ -> [_ w470]
        tunnel: [w459 w467] -> _
        tunnel: _ -> [_ w466]
        tunnel: [_ w460] -> _
        tunnel: [_ w464] -> _
        tunnel: [_ w462] -> _
        tunnel: [_ TRUE] -> _
        frame False {
        }
        frame True {
          n136 = call-poly <vilib>:"NI VeriStand - Search for Item.vi"("error in"=w469, "Item GUID"=w470, "Section Ref in"=w471) -> ("error out"=w468:errorcluster, "Item Refs"=w460:T2[])  [unwired: 5 in, 2 out]
          n137 = call <vilib>:"NI VeriStand - Get Channel Block Data References.vi"("error in (no error)"=w468, "Access"=Data_Access_Type."Write", "Channel Refs"=w460, "Device Ref in"=w466) -> ("error out"=w467:errorcluster, "Values Array"=w463:dbl[], "Block Data Refs"=w464:T8[])  [unwired: 4 in, 1 out]
          n138 = To Unsigned Word Integer(number=w463) -> (unsigned 16bit integer=w462:u16[])
        }
      }
    }
    frame Enabled {
    }
  }
